vi "StartTraceGUIvi.vi"(8 "Error In":errorcluster) -> (0 "Error Out":errorcluster)   [LabVIEW 2018]
uses:
  TracerLibrary/Tracer/Tracer.lvclass
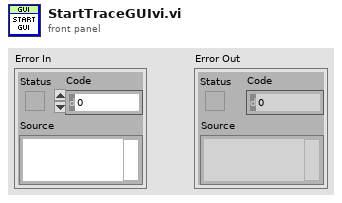
[diagram p1: front panel]
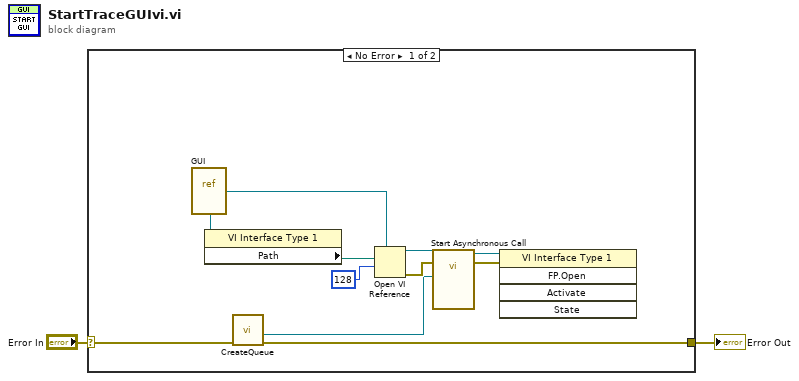
[diagram p0: block diagram]
diagram:
  n1 = case shown="No Error" "Error In" {
    selector: "Error In" -> [w10 w13]
    tunnel: [w9 w13] -> w1
    frame No Error {
      n2 = vi-ref "GUI.vi"() -> (w5:refnum<vi>)
      n3 = property class="VI Interface Type 1"(reference=w5) -> ("Path"=w8:path)  [unwired: 1 in, 2 out]
      n4 = call "CreateQueue.vi"("Error In"=w10) -> ("Error Out"=w9:errorcluster, "Trace Out"=w3:refnum<queue>)  [unwired: 9 in]
      n5 = Open VI Reference(type specifier VI Refnum (for type only)=w5, vi path=w8, options=128) -> (vi reference=w6:refnum<vi>, error out=w11:errorcluster)  [unwired: 3 in]
      n6 = call-by-ref "Start Asynchronous Call"(reference=w6, error in=w11, "TraceQueue"=w3) -> (reference out=w4:refnum<vi>, error out=w12:errorcluster)  [unwired: 11 in]
      n7 = invoke class="VI Interface Type 1" method="FP.Open"(reference=w4, error in=w12) -> ()  [unwired: 3 in, 5 out]
    }
    frame Error {
    }
  }
  "Error Out" <- w1
